vi "Equipstate~dialog.vi"() -> (1 "RecordDate":string, 2 "Equipstate":string)   [LabVIEW 2020, in "设备状态接口.lvlib"]
uses:
  Equipstate.ctl
panel:
  in  "FAULT":bool
  in  "PLAN_STANDBY":bool
  in  "ABNORMAL_ENVIRON":bool
  in  "ABNORMAL_INFO":bool
  in  "ABNORMAL_QUALITY":bool
  in  "PROCESS_INSPECTION":bool
  in  "ABNORMAL_BLOCKING":bool
  in  "REFUELLING":bool
  in  "ABNORMAL_INCOMING":bool
  in  "确定":bool
  in  "Equipstate":T1
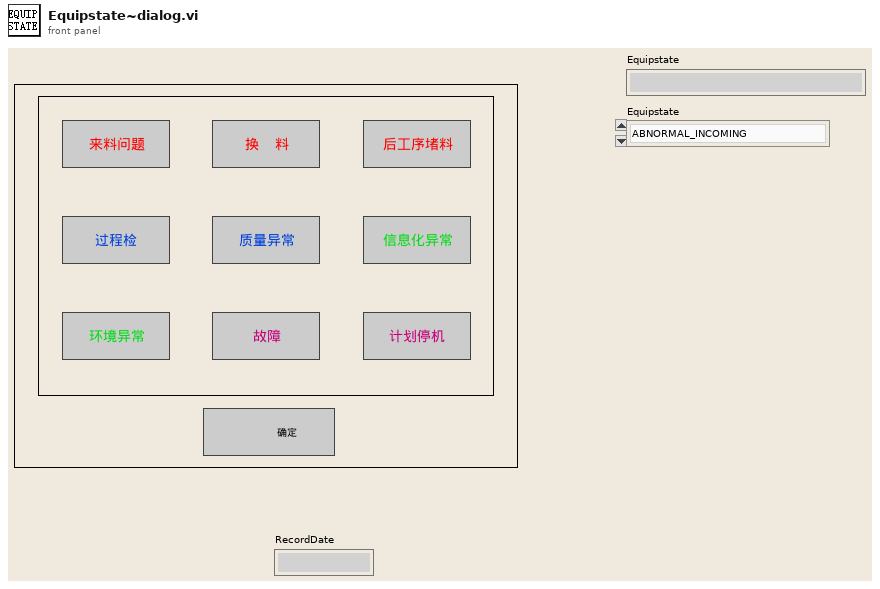
[diagram p1: front panel]
types:
  T1 = typedef "设备状态接口.lvlib/Equipstate.ctl" = enum16{"ABNORMAL_INCOMING", "REFUELLING", "ABNORNAL_BLOCKING", "PROCESS_INSPECTION", "ABNORMAL_QUALITY", "ABNORMAL_INFO", "ABNORMAL_ENVIRON", "PLAN_STANDBY"}
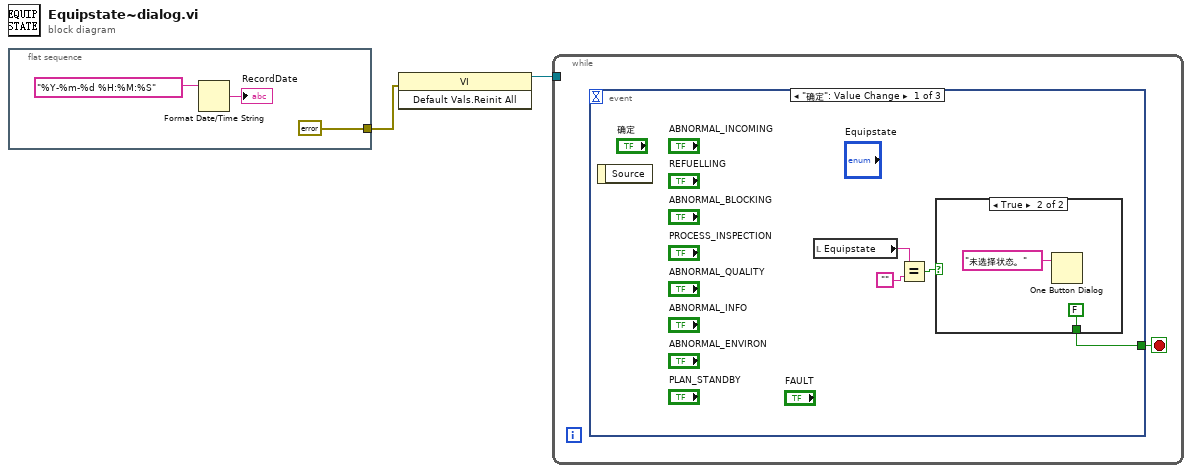
[diagram p0: block diagram]
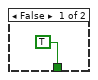
[diagram p2: hidden frame]
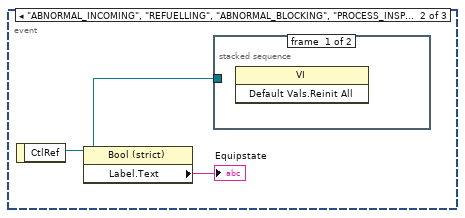
[diagram p3: hidden frame]
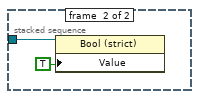
[diagram p4: hidden frame]
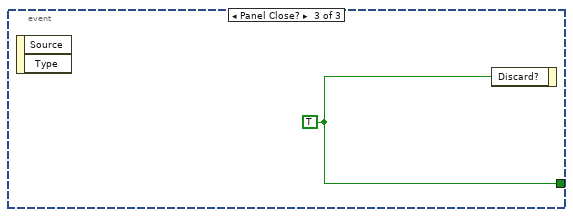
[diagram p5: hidden frame]
diagram:
  n1 = flat-sequence {
    tunnel: [errorcluster {"status"=FALSE, "code"=0, "source"=""} ("错误常量")] -> w1
    frame #0 {
      n2 = Format Date/Time String(time format string (%c)="%Y-%m-%d %H:%M:%S" ("时间格式字符串(%c)")) -> (date/time string=→"RecordDate":string)  [unwired: 2 in]
    }
  }
  n3 = invoke class="VI" method="Default Vals.Reinit All"(error in=w1) -> (reference out=w2:refnum<vi>)  [unwired: 2 in, 2 out]
  n4 = while {
    tunnel: w2 -> [_]
    stop <- w6 stop-if-true
    n5 = event shown="[0] \"确定\": Value Change" {
      selector: _ -> [_ _ _]
      dyn-events: _ -> [_ _ _]
      timeout: _ -> [_ _ _]
      tunnel: [w7 _ w18] -> w6
      event "确定": Value Change {
        n6 = event-data() -> ()  [unwired: 1 in, 1 out]
        n7 = local read "Equipstate"() -> (w10:string)
        n8 = Equal?(x=w10, y="") -> (x = y?=w8:bool)
        n9 = case shown="True" w8 {
          tunnel: [TRUE FALSE] -> w7
          frame False {
          }
          frame True {
            n10 = One Button Dialog(message="未选择状态。" ("消息")) -> ()  [unwired: 1 in, 1 out]
          }
        }
      }
      event "ABNORMAL_INCOMING", "REFUELLING", "ABNORMAL_BLOCKING", "PROCESS_INSPECTION", "ABNORMAL_QUALITY", "ABNORMAL_INFO", "ABNORMAL_ENVIRON", "PLAN_STANDBY", "FAULT": Value Change {
        n11 = event-data() -> ("CtlRef"=w14:refnum<vi>)  [unwired: 1 in]
        n12 = property class="Bool (strict)"(reference=w14) -> ("Label.Text"=→"Equipstate":string)  [unwired: 1 in, 2 out]
        n13 = stacked-sequence {
          tunnel: w14 -> [_ w17]
          frame #0 {
            n14 = invoke class="VI" method="Default Vals.Reinit All"() -> ()  [unwired: 3 in, 3 out]
          }
          frame #1 {
            n15 = property class="Bool (strict)"(reference=w17, "Value"=TRUE) -> ()  [unwired: 1 in, 2 out]
          }
        }
      }
      event Panel Close? {
        w18 = TRUE
        n16 = event-data() -> ()  [unwired: 1 in, 2 out]
        n17 = event-data("Discard?"=w18) -> ()  [unwired: 1 in, 1 out]
      }
    }
  }
